vi "FTW-JSON-LexicalScan-Digits.vi"(0 "JSON String":T1, 11 "error in":errorcluster) -> (4 "JSON String Out":T1, 8 "Digits":u8[](array[numeric]), 15 "error out":errorcluster)   [LabVIEW 2015]
uses:
  FTW-JSON-LexicalScan.ctl
  FTW-JSON-LexicalScan-Char.vi
panel:
  # "Inputs"
  # "Outputs"
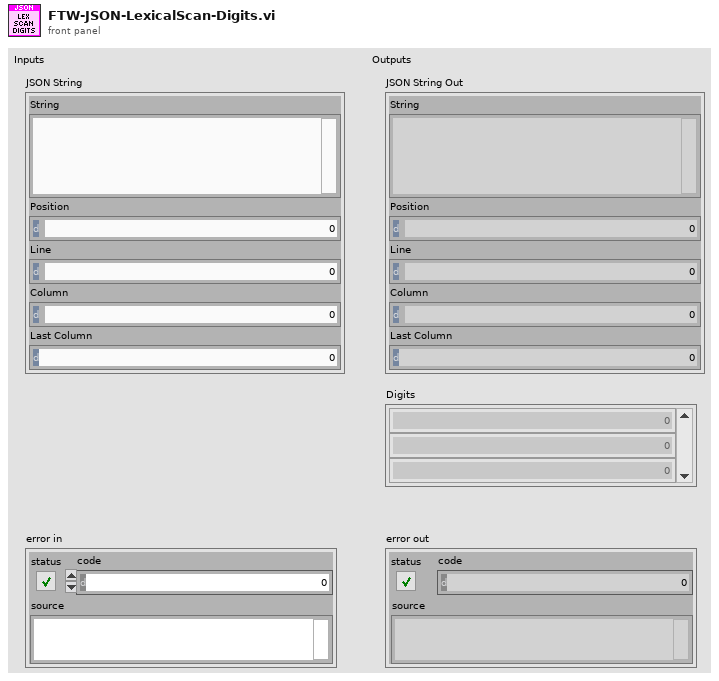
[diagram p1: front panel]
types:
  T1 = typedef "FTW-JSON-LexicalScan.ctl" = cluster{"String":string, "Position":i32, "Line":i32, "Column":i32, "Last Column":i32}
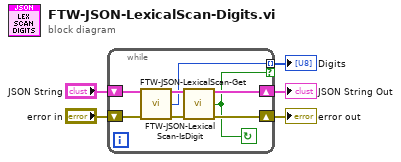
[diagram p0: block diagram]
diagram:
  n1 = while {
    shift-right: [w10] -> w2
    shift-left: "error in" -> [w13]
    shift-right: [w8] -> w3
    shift-left: "JSON String" -> [w11]
    tunnel: [w7] -> w1 mode=indexing if=w6
    stop <- w6 continue-if-true
    n2 = call "FTW-JSON-LexicalScan-Get.vi"("JSON String"=w11, "error in"=w13) -> ("JSON String Out"=w9:T1, "Char"=w7:u8, "error out"=w12:errorcluster)  [unwired: 11 in]
    n3 = call "FTW-JSON-LexicalScan-IsDigit.vi"("JSON String"=w9, "error in"=w12) -> ("JSON String Out"=w8:T1, "Is Digit"=w6:bool, "error out"=w10:errorcluster)  [unwired: 11 in]
  }
  "Digits" <- w1
  "error out" <- w2
  "JSON String Out" <- w3
